vi "visComClientUI.vi"(10 "Plugin Info":T3, 11 "ConnectionData":T4) -> ()   [LabVIEW 2016]
uses:
  General/RemoteFiles/connectionData.ctl
  General/CorePluginInfo.ctl
  Controls/visionData.ctl
panel:
  out "Image":T1(plugin-control)
  out "DataPacket":T2
  in  "Update rate":dbl
  out "Array":string[](array[string])
  in  "Make request":bool
  in  "Request type":T5(ring)
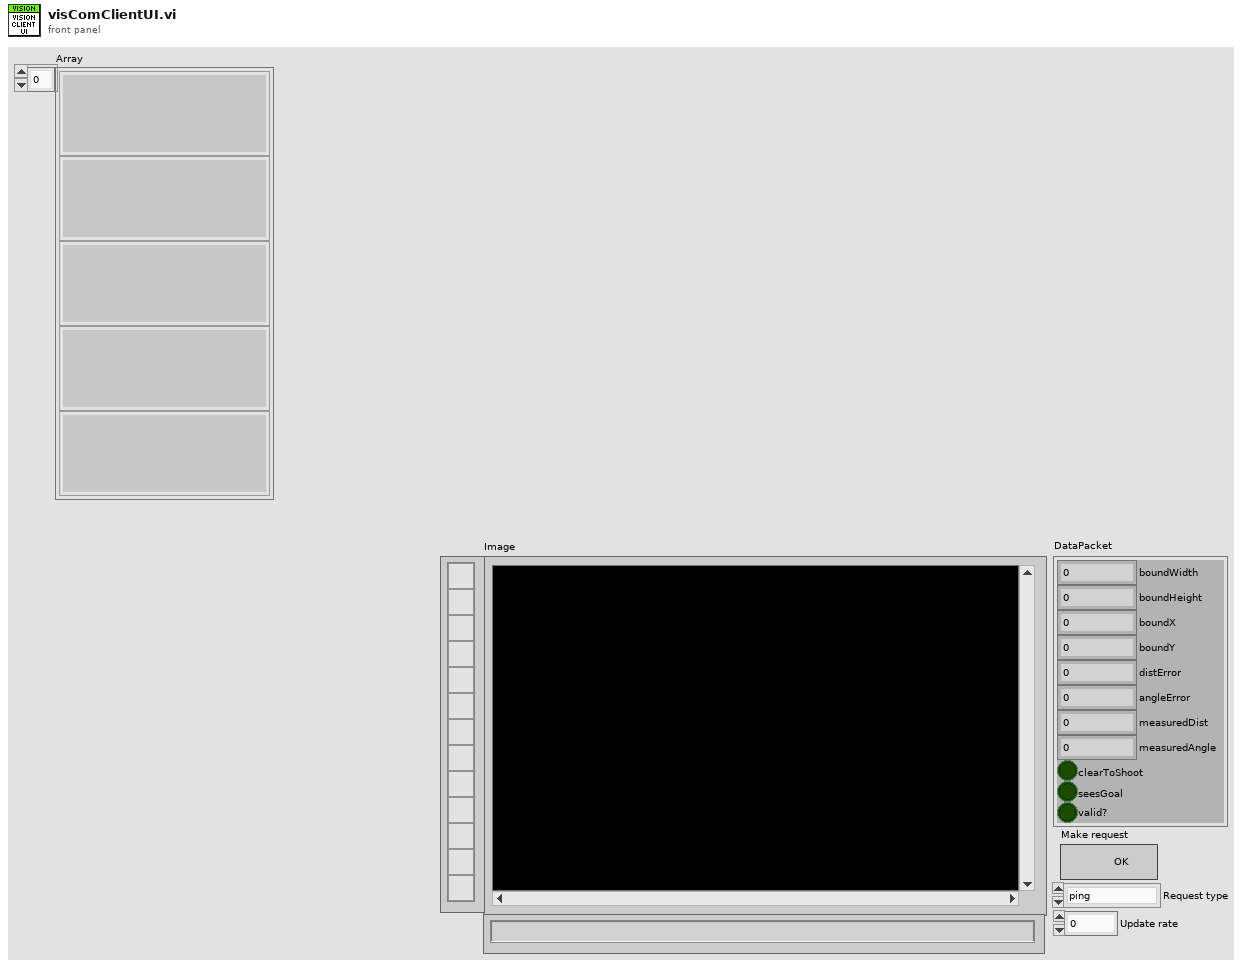
[diagram p1: front panel]
types:
  T1 = typedef "IMAQ Image.ctl" = refnum<image>
  T2 = typedef "visionData.ctl" = cluster{"boundWidth":dbl, "boundHeight":dbl, "boundX":dbl, "boundY":dbl, "distError":dbl, "angleError":dbl, "measuredDist":dbl, "measuredAngle":dbl, "clearToShoot":bool, "seesGoal":bool, "valid?":bool}
  T3 = typedef "CorePluginInfo.ctl" = cluster{"Notifiers":cluster{"Robot IP Notifier":refnum<notifier>, "Window Mode Notifier":refnum<notifier>, "Stop Notifier":refnum<notifier>}}
  T4 = typedef "connectionData.ctl" = cluster{"host":string, "user":string, "password":string, "port":u16}
  T5 = enum16{"ping", "raw frame", "masked frame", "data"}
  T6 = typedef "Image Type" = u32
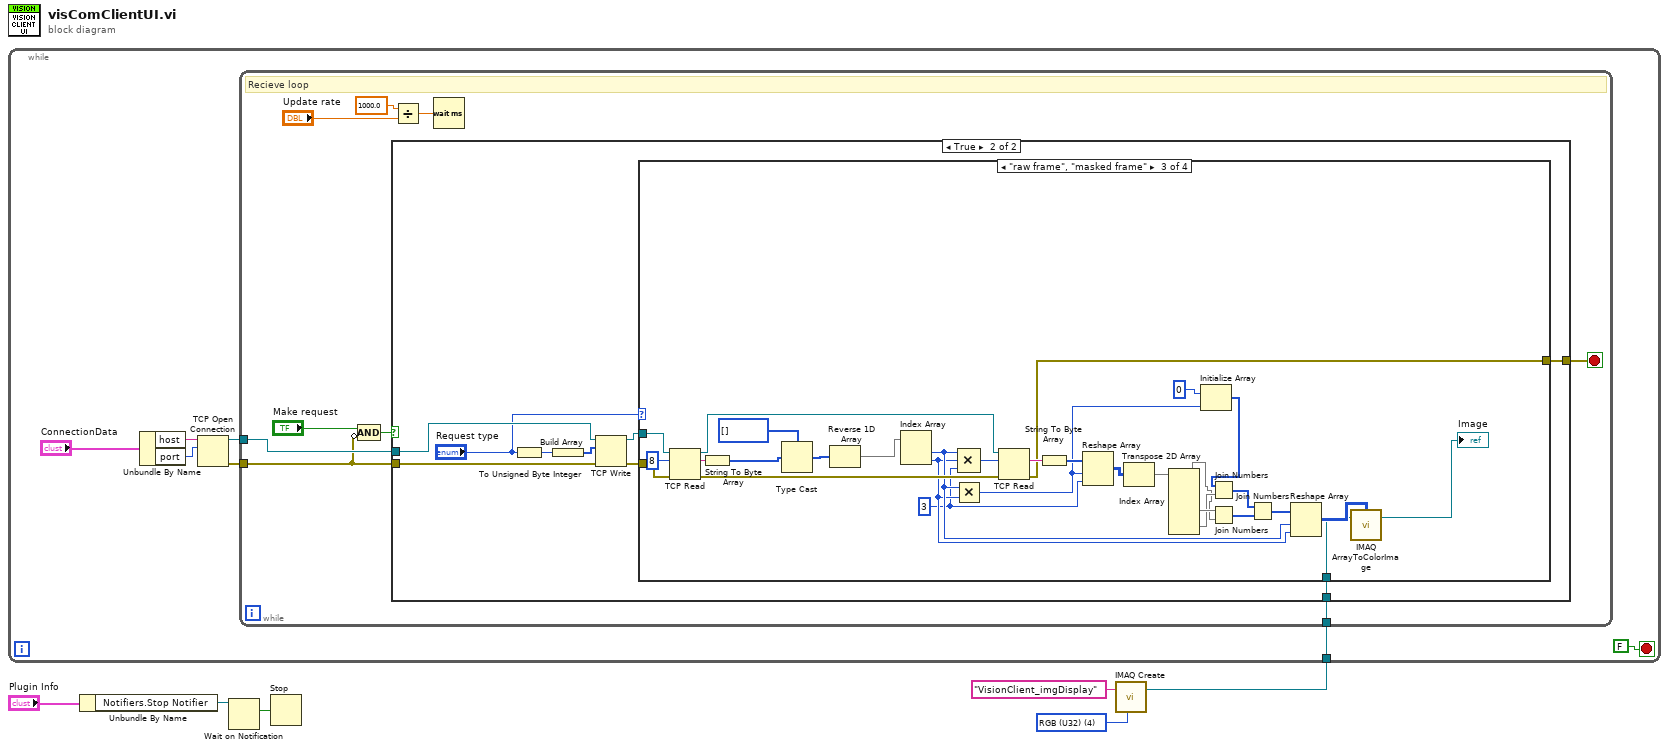
[diagram p0: block diagram]
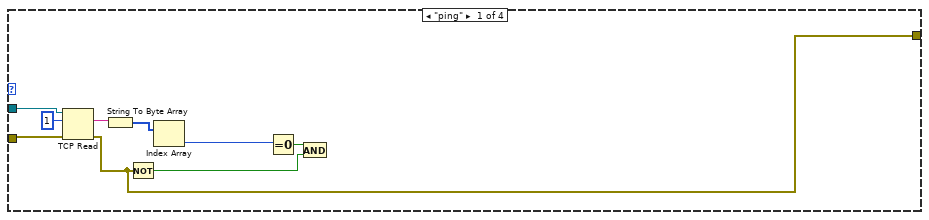
[diagram p3: hidden frame]
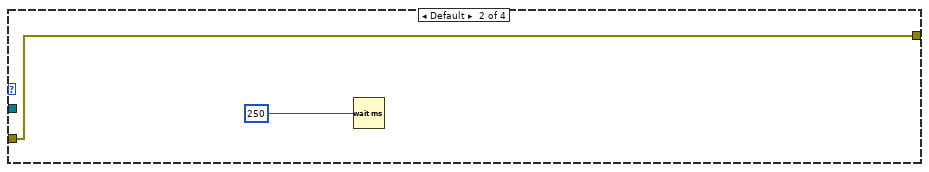
[diagram p4: hidden frame]
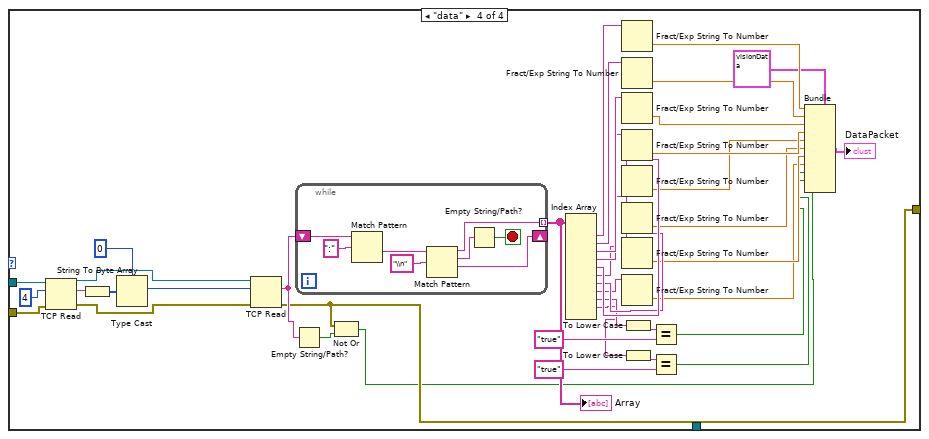
[diagram p5: hidden frame]
diagram:
  w2 = T6 4 items=["Grayscale (U8)", "Grayscale (I16)", "Grayscale (SGL)", "Complex (CSG)", "RGB (U32)", "HSL (U32)", "RGB (U64)", "Grayscale (U16)"] ("Image Type")
  n1 = Unbundle By Name("Plugin Info") -> ("Notifiers.Stop Notifier"=w5:refnum<notifier>)
  n2 = Wait on Notification(notifier=w5) -> (notification=w4:bool)  [unwired: 3 in, 3 out]
  n3 = Stop(stop? (T)=w4) -> ()
  n4 = call "IMAQ Create"("Image Name"="VisionClient_imgDisplay", "Image Type"=w2) -> ("New Image"=w1:T1)  [unwired: 3 in, 1 out]
  n5 = while {
    tunnel: w1 -> [w7]
    stop <- FALSE stop-if-true
    n6 = Unbundle By Name("ConnectionData") -> ("host"=w11:string, "port"=w10:u16)
    n7 = TCP Open Connection(address=w11, remote port or service name=w10) -> (connection ID=w13:refnum<k5>, error out=w9:errorcluster)  [unwired: 3 in]
    n8 = while {
      tunnel: w13 -> [w22]
      tunnel: w9 -> [w16]
      tunnel: w7 -> [w14]
      stop <- w21 stop-if-true
      # "Recieve loop"
      n9 = Compound Arithmetic op=AND("Make request", invert w16) -> (w15:bool)
      n10 = case shown="True" w15 {
        tunnel: w22 -> [_ w32]
        tunnel: w16 -> [w23 w28]
        tunnel: [w23 w25] -> w21
        tunnel: w14 -> [_ w24]
        frame False {
        }
        frame True {
          n11 = To Unsigned Byte Integer(number="Request type") -> (unsigned 8bit integer=w27:u8)
          n12 = Build Array(w27) -> (w26:u8[])
          n13 = TCP Write(connection ID=w32, data in=w26, error in (no error)=w28) -> (connection ID out=w30:refnum<k5>, error out=w29:errorcluster)  [unwired: 1 in, 1 out]
          n14 = case shown="\"raw frame\", \"masked frame\"" "Request type" {
            tunnel: w30 -> [w41 _ w58 w114]
            tunnel: w29 -> [w34 w43 w57 w106]
            tunnel: [w33 w43 w56 w77] -> w25
            tunnel: w24 -> [_ _ w44 _]
            frame "ping" {
              n15 = TCP Read(connection ID=w41, bytes to read=1, error in (no error)=w34) -> (data out=w39:string, error out=w33:errorcluster)  [unwired: 2 in, 1 out]
              n16 = String To Byte Array(string=w39) -> (unsigned byte array=w38:u8[])
              n17 = Not(x=w33) -> (.not. x?=w35:bool)
              n18 = Index Array(array=w38) -> (element=w37:u8)  [unwired: 1 in]
              n19 = Equal To 0?(x=w37) -> (x = 0?=w36:bool)
              n20 = And(x=w36, y=w35) -> ()  [unwired: 1 out]
            }
            frame Default {
              n21 = Wait (ms)(milliseconds to wait=u32 250) -> ()  [unwired: 1 out]
            }
            frame "raw frame", "masked frame" {
              w63 = 3 ("value")
              n22 = TCP Read(connection ID=w58, bytes to read=8, error in (no error)=w57) -> (connection ID out=w69:refnum<k5>, data out=w73:string, error out=w68:errorcluster)  [unwired: 2 in]
              n23 = String To Byte Array(string=w73) -> (unsigned byte array=w72:u8[])
              n24 = Type Cast(type=i32[] [], x=w72) -> (*(type *) &x=w48:i32[])
              n25 = Reverse 1D Array(array=w48) -> (reversed array=w47:i32[])
              n26 = Index Array(array=w47) -> (element #1=w65:i32, element #2=w64:i32)  [unwired: 2 in]
              n27 = Multiply(x=w65, y=w64) -> (x*y=w55:i32)
              n28 = Compound Arithmetic op=MULTIPLY(w65, w64, w63) -> (w70:i32)
              n29 = TCP Read(connection ID=w69, bytes to read=w70, error in (no error)=w68) -> (data out=w67:string, error out=w56:errorcluster)  [unwired: 2 in, 1 out]
              n30 = String To Byte Array(string=w67) -> (unsigned byte array=w62:u8[])
              n31 = Reshape Array(w62, w55, w63) -> (w50:u8[][])
              n32 = Transpose 2D Array(2D array=w50) -> (transposed array=w49:u8[][])
              n33 = Index Array(array=w49) -> (element #1=w51:u8[], element #2=w61:u8[], element #3=w52:u8[])  [unwired: 6 in]
              n34 = Initialize Array(u8 0, w55) -> (w53:u8[])
              n35 = Join Numbers(hi=w53, lo=w52) -> ((hi.lo)=w59:u16[])
              n36 = Join Numbers(hi=w61, lo=w51) -> ((hi.lo)=w60:u16[])
              n37 = Join Numbers(hi=w59, lo=w60) -> ((hi.lo)=w66:u32[])
              n38 = Reshape Array(w66, w65, w64) -> (w46:u32[][])
              n39 = call "IMAQ ArrayToColorImage"("Image Pixels (U32)"=w46, "Image"=w44) -> ("Image Out"=→"Image":T1)  [unwired: 3 in, 1 out]
            }
            frame "data" {
              n40 = TCP Read(connection ID=w114, bytes to read=4, error in (no error)=w106) -> (connection ID out=w108:refnum<k5>, data out=w112:string, error out=w107:errorcluster)  [unwired: 2 in]
              n41 = String To Byte Array(string=w112) -> (unsigned byte array=w111:u8[])
              n42 = Type Cast(type=0, x=w111) -> (*(type *) &x=w109:i32)
              n43 = TCP Read(connection ID=w108, bytes to read=w109, error in (no error)=w107) -> (data out=w79:string, error out=w77:errorcluster)  [unwired: 2 in, 1 out]
              n44 = Empty String/Path?(string/path=w79) -> (empty?=w78:bool)
              n45 = while {
                shift-right: [w118] -> _
                shift-left: w79 -> [w122]
                tunnel: [w115] -> w102 mode=indexing
                stop <- w116 stop-if-true
                n46 = Match Pattern(string=w122, regular expression=":") -> (after substring=w120:string)  [unwired: 1 in, 3 out]
                n47 = Match Pattern(string=w120, regular expression="\\n") -> (before substring=w115:string, match substring=w117:string, after substring=w118:string)  [unwired: 1 in, 1 out]
                n48 = Empty String/Path?(string/path=w117) -> (empty?=w116:bool)
              }
              "Array" <- w102
              n49 = Not Or(1:w78, 2:w77) -> (0:w76:bool)
              n50 = Index Array(array=w102) -> (element #1=w100:string, element #2=w105:string, element #3=w99:string, element #4=w98:string, element #5=w95:string, element #6=w94:string, element #7=w93:string, element #8=w92:string, element #9=w87:string, element #10=w81:string)  [unwired: 11 in, 1 out]
              n51 = Fract/Exp String To Number(string=w100) -> (number=w104:dbl)  [unwired: 3 in, 1 out]
              n52 = Fract/Exp String To Number(string=w105) -> (number=w103:dbl)  [unwired: 3 in, 1 out]
              n53 = Fract/Exp String To Number(string=w99) -> (number=w97:dbl)  [unwired: 3 in, 1 out]
              n54 = Fract/Exp String To Number(string=w98) -> (number=w96:dbl)  [unwired: 3 in, 1 out]
              n55 = Fract/Exp String To Number(string=w95) -> (number=w91:dbl)  [unwired: 3 in, 1 out]
              n56 = Fract/Exp String To Number(string=w94) -> (number=w90:dbl)  [unwired: 3 in, 1 out]
              n57 = Fract/Exp String To Number(string=w93) -> (number=w89:dbl)  [unwired: 3 in, 1 out]
              n58 = Fract/Exp String To Number(string=w92) -> (number=w88:dbl)  [unwired: 3 in, 1 out]
              n59 = To Lower Case(string=w87) -> (all lower case string=w86:string)
              n60 = To Lower Case(string=w81) -> (all lower case string=w82:string)
              n61 = Equal?(x=w86, y="true") -> (x = y?=w84:bool)
              n62 = Equal?(x=w82, y="true") -> (x = y?=w80:bool)
              n63 = Bundle(cluster=T2 {"boundWidth"=0.0, "boundHeight"=0.0, "boundX"=0.0, "boundY"=0.0, "distError"=0.0, "angleError"=0.0, "measuredDist"=0.0, "measuredAngle"=0.0, "clearToShoot"=FALSE, "seesGoal"=FALSE, "valid?"=FALSE} ("DataPacket"), "boundWidth"=w104, "boundHeight"=w103, "boundX"=w97, "boundY"=w96, "distError"=w91, "angleError"=w90, "measuredDist"=w89, "measuredAngle"=w88, "clearToShoot"=w84, "seesGoal"=w80, "valid?"=w76) -> (→"DataPacket":T2)
            }
          }
        }
      }
      n64 = Divide(x=1000.0, y="Update rate") -> (x/y=w18:dbl)
      n65 = Wait (ms)(milliseconds to wait=w18) -> ()  [unwired: 1 out]
    }
  }
